vi "SubVI Tester.vi"() -> ()   [LabVIEW 2017]
panel:
  in  "Weather Data In":T1={"Current Temperature"=0.0, "Max Temperature"=0.0, "Min Temperature"=0.0, "Warning?"=FALSE, "Warning Text"="No Warning"}
  in  "Min Temperature":dbl=10.0
  in  "Max Temperature":dbl=30.0
  in  "Stop":bool
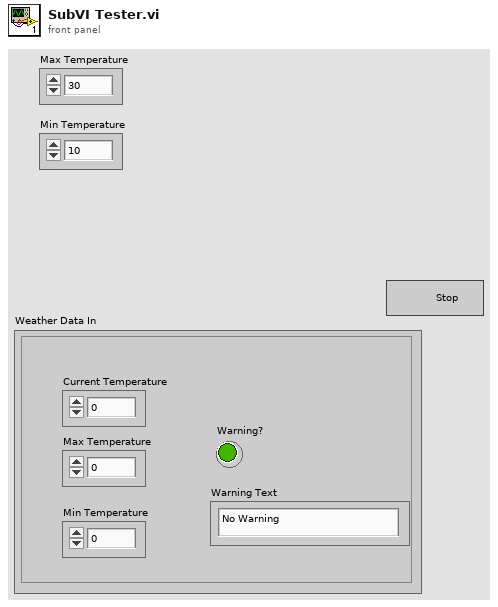
[diagram p1: front panel]
types:
  T1 = cluster{"Current Temperature":dbl, "Max Temperature":dbl, "Min Temperature":dbl, "Warning?":bool, "Warning Text":string}
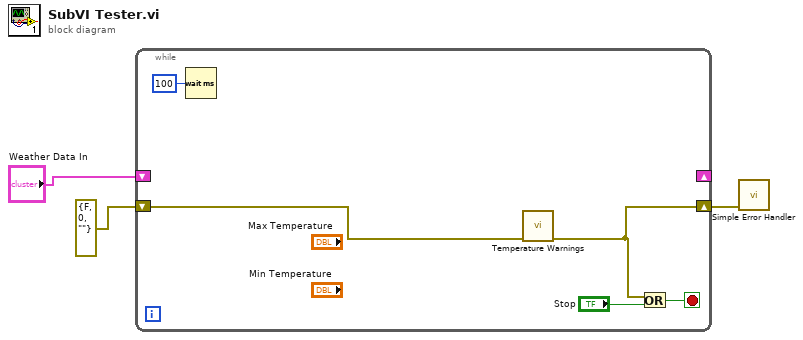
[diagram p0: block diagram]
diagram:
  n1 = while {
    shift-right: [w5] -> w3
    shift-left: errorcluster {"status"=FALSE, "code"=0, "source"=""} ("error in") -> [w4]
    shift-right: _ -> [_]
    shift-left: "Weather Data In" -> [_]
    stop <- w6 stop-if-true
    n2 = Wait (ms)(milliseconds to wait=u32 100) -> ()  [unwired: 1 out]
    n3 = call "Temperature Warnings.vi"("Error In"=w4) -> ("Error Out"=w5:errorcluster)  [unwired: 9 in, 1 out]
    n4 = Or(x=w5, y="Stop") -> (x .or. y?=w6:bool)
  }
  n5 = call <vilib>:"Simple Error Handler.vi"("error in (no error)"=w3) -> ()  [unwired: 4 in, 5 out]
